vi "RS232C_Cmd_G_OK_re.vi"(4 "Main/Sub":bool=TRUE, 5 "Delimiter":string="\\r\\n", 6 "Command String":string, 7 "PortNumber":i32) -> (0 "OK Done":bool, 1 "Received String3":string, 2 "Received String2":string, 3 "Received String1":string)   [LabVIEW 2016]
panel:
  # "Port Number 0=COM1"
  # "Send 'Command String', (receive 'OK'), send 'G Command' (and receive 'OK')."
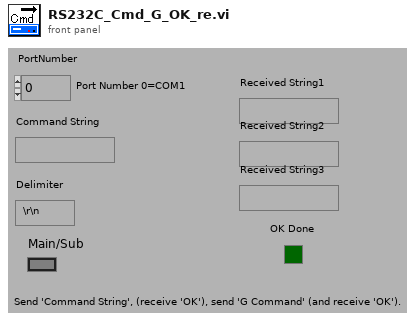
[diagram p1: front panel]
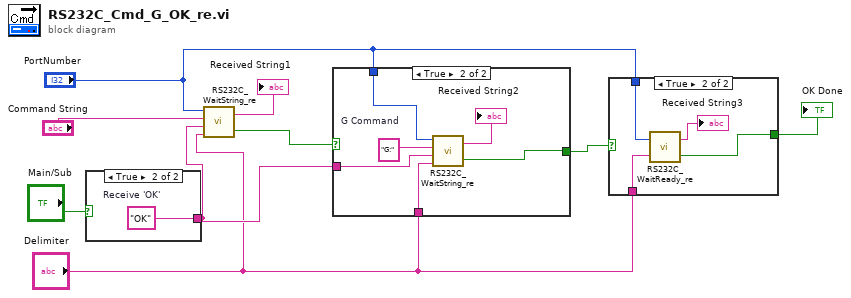
[diagram p0: block diagram]
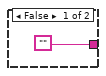
[diagram p2: hidden frame]
diagram:
  n1 = case shown="True" "Main/Sub" {
    tunnel: ["" w11] -> w2
    frame False {
    }
    frame True {
      w11 = "OK"  # Receive 'OK'
    }
  }
  n2 = call "RS232C_WaitString_re.vi"("Delimiter"="Delimiter", "String to Receive"=w2, "String to Send"="Command String", "PortNumber"="PortNumber") -> ("OK Done"=w4:bool, "String Received"=→"Received String1":string)
  n3 = case shown="True" w4 {
    selector: w4 -> [w12 _]
    tunnel: "PortNumber" -> [_ w18]
    tunnel: [w12 w15] -> w8
    tunnel: w2 -> [_ w14]
    tunnel: "Delimiter" -> [_ w13]
    frame False {
    }
    frame True {
      w17 = "G:"  # G Command
      n4 = call "RS232C_WaitString_re.vi"("Delimiter"=w13, "String to Receive"=w14, "String to Send"=w17, "PortNumber"=w18) -> ("OK Done"=w15:bool, "String Received"=→"Received String2":string)
    }
  }
  n5 = case shown="True" w8 {
    selector: w8 -> [w19 _]
    tunnel: "PortNumber" -> [_ w22]
    tunnel: [w19 w23] -> w9
    tunnel: "Delimiter" -> [_ w20]
    frame False {
    }
    frame True {
      n6 = call "RS232C_WaitReady_re.vi"("Delimiter"=w20, "PortNumber"=w22) -> ("OK Done"=w23:bool, "String Received"=→"Received String3":string)
    }
  }
  "OK Done" <- w9
